vi "Simula DI.vi"(10 "statoDO_cDaq":T2) -> (2 "Stato DI_Cdaq":T1)   [LabVIEW 2019]
uses:
  controls/statoDO_Cdaq.ctl
panel:
  in  "Pulsante Start prova":bool
  in  "Elettoserrature chiuse":bool=TRUE
  in  "Rot bloccato (0=bloccato)":bool
  in  "Reset allarme":bool
  in  "Stop prova":bool
  in  "Inverter mot freno pronto":bool=TRUE
  in  "AFE aliment DC pronto":bool=TRUE
  in  "AFE aliment AC pronto":bool=TRUE
  in  "Centralina sicurezza ok":bool=TRUE
  in  "Interrutt generale chiuso":bool=TRUE
  # "FORZA DI"
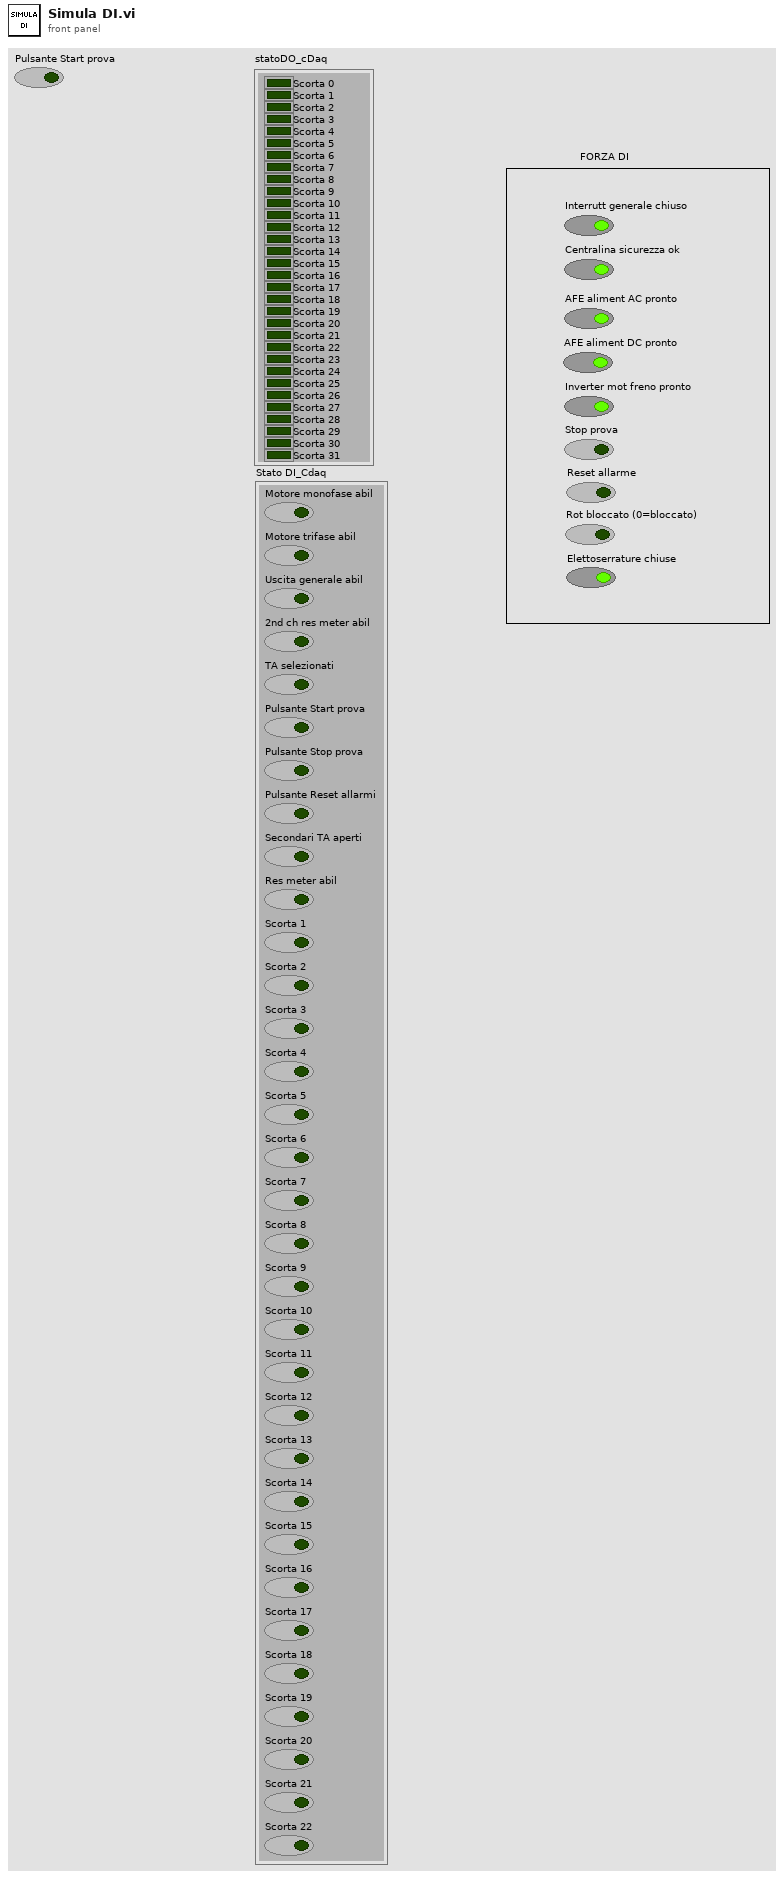
[diagram p1: front panel]
types:
  T1 = cluster{"Motore monofase abil":bool, "Motore trifase abil":bool, "Uscita generale abil":bool, "2nd ch res meter abil":bool, "TA selezionati":bool, "Pulsante Start prova":bool, "Pulsante Stop prova":bool, "Pulsante Reset allarmi":bool, "Secondari TA aperti":bool, "Res meter abil":bool, "Scorta 1":bool, "Scorta 2":bool, "Scorta 3":bool, "Scorta 4":bool, "Scorta 5":bool, "Scorta 6":bool, "Scorta 7":bool, "Scorta 8":bool, "Scorta 9":bool, "Scorta 10":bool, "Scorta 11":bool, "Scorta 12":bool, "Scorta 13":bool, "Scorta 14":bool, "Scorta 15":bool, "Scorta 16":bool, "Scorta 17":bool, "Scorta 18":bool, "Scorta 19":bool, "Scorta 20":bool, "Scorta 21":bool, "Scorta 22":bool}
  T2 = typedef "statoDO_Cdaq.ctl" = cluster{"Scorta 0":bool, "Scorta 1":bool, "Scorta 2":bool, "Scorta 3":bool, "Scorta 4":bool, "Scorta 5":bool, "Scorta 6":bool, "Scorta 7":bool, "Scorta 8":bool, "Scorta 9":bool, "Scorta 10":bool, "Scorta 11":bool, "Scorta 12":bool, "Scorta 13":bool, "Scorta 14":bool, "Scorta 15":bool, "Scorta 16":bool, "Scorta 17":bool, "Scorta 18":bool, "Scorta 19":bool, "Scorta 20":bool, "Scorta 21":bool, "Scorta 22":bool, "Scorta 23":bool, "Scorta 24":bool, "Scorta 25":bool, "Scorta 26":bool, "Scorta 27":bool, "Scorta 28":bool, "Scorta 29":bool, "Scorta 30":bool, "Scorta 31":bool}
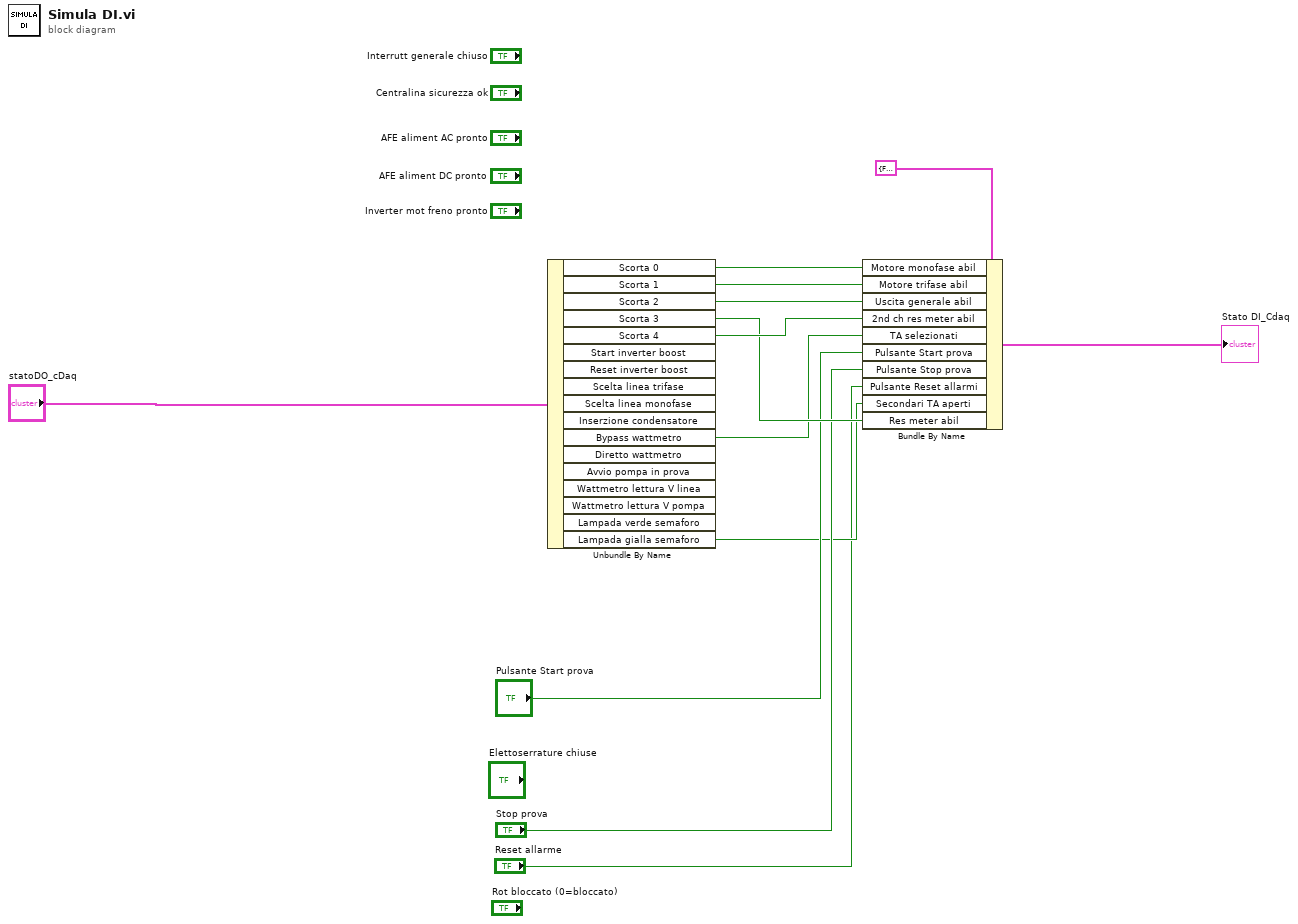
[diagram p0: block diagram]
diagram:
  n1 = Unbundle By Name("statoDO_cDaq") -> ("Scorta 0"=w10:bool, "Scorta 1"=w9:bool, "Scorta 2"=w8:bool, "Scorta 3"=w6:bool, "Scorta 4"=w7:bool, "Bypass wattmetro"=w5:bool, "Lampada gialla semaforo"=w2:bool)  [unwired: 10 out]
  n2 = Bundle By Name(cluster=T1 {"Motore monofase abil"=FALSE, "Motore trifase abil"=FALSE, "Uscita generale abil"=FALSE, "2nd ch res meter abil"=FALSE, "TA selezionati"=FALSE, "Pulsante Start prova"=FALSE, "Pulsante Stop prova"=FALSE, "Pulsante Reset allarmi"=FALSE, "Secondari TA aperti"=FALSE, "Res meter abil"=FALSE, "Scorta 1"=FALSE, "Scorta 2"=FALSE, "Scorta 3"=FALSE, "Scorta 4"=FALSE, "Scorta 5"=FALSE, "Scorta 6"=FALSE, "Scorta 7"=FALSE, "Scorta 8"=FALSE, "Scorta 9"=FALSE, "Scorta 10"=FALSE, "Scorta 11"=FALSE, "Scorta 12"=FALSE, "Scorta 13"=FALSE, "Scorta 14"=FALSE, "Scorta 15"=FALSE, "Scorta 16"=FALSE, "Scorta 17"=FALSE, "Scorta 18"=FALSE, "Scorta 19"=FALSE, "Scorta 20"=FALSE, "Scorta 21"=FALSE, "Scorta 22"=FALSE} ("Stato DI_Cdaq 2"), "Motore monofase abil"=w10, "Motore trifase abil"=w9, "Uscita generale abil"=w8, "2nd ch res meter abil"=w7, "TA selezionati"=w5, "Pulsante Start prova"="Pulsante Start prova", "Pulsante Stop prova"="Stop prova", "Pulsante Reset allarmi"="Reset allarme", "Secondari TA aperti"=w2, "Res meter abil"=w6) -> (→"Stato DI_Cdaq":T1)
